vi "isSessionRefValid.vi"(11 "Client in":refnum<class "Client.lvclass">) -> (2 "Session ref valid":bool, 3 "Client out":refnum<class "Client.lvclass">)   [LabVIEW 2013, in "MQTT Client.lvlib" / "Client.lvclass"]
uses:
  Client.lvclass
  Client.lvclass/Client.ctl
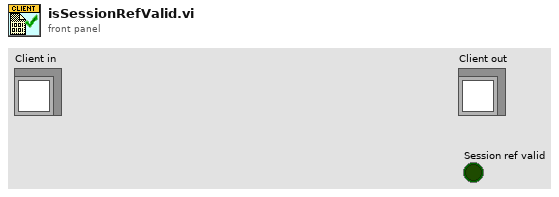
[diagram p1: front panel]
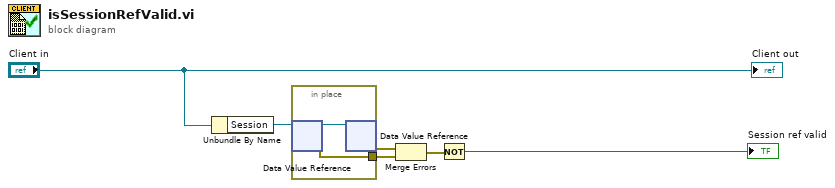
[diagram p0: block diagram]
diagram:
  n1 = Unbundle By Name("Client in") -> ("Session"=w4:refnum<data-value>)
  n2 = in-place {
    in-place-border: [w7] -> w2
    n3 = in-place-dvr #1(w4) -> (w8:refnum<class "Session.Client.lvclass">, w7:errorcluster)
    n4 = in-place-dvr #1(w8) -> (w3:errorcluster)  [unwired: 1 out]
  }
  n5 = Merge Errors(w3, w2) -> (w1:errorcluster)
  n6 = Not(x=w1) -> (.not. x?=→"Session ref valid":bool)
  "Client out" <- "Client in"
